vi "play-AFM-CS-imaging_v4.vi"() -> ()   [LabVIEW 2017]
uses:
  controls/boolean_info.ctl
  controls/TF-params.ctl
  controls/z-axis-params_v4_prescan.ctl
  <userlib>/_matio/level5/Public/MAT-File Data Types.ctl
  <vilib>/userdefined/High Color/nirio_resource_hc.ctl
  controls/expMetaData_prescan.ctl
  <vilib>/Utility/file.llb/Read Delimited Spreadsheet (DBL).vi
  <vilib>/FPGAPlugInAG/cRIO-9082/niLvFpga_Open_cRIO-9082.vi
  <vilib>/rvi/interface/common/dynamic/niFpgaDynamicAddResources.vi
  <vilib>/FPGAPlugInAG/Dynamic/niLvFpga_Reset_Dynamic.vi
  <vilib>/rvi/interface/common/niFpgaWaitOnOcc.vi
  <vilib>/Utility/error.llb/Error Cluster From Error Code.vi
  <vilib>/rvi/errors/niLvFpgaAdjustHostInterfaceError.vi
  <vilib>/FPGAPlugInAG/Dynamic/niLvFpga_Run_Dynamic.vi
  <vilib>/Utility/file.llb/Write Delimited Spreadsheet (DBL).vi
  <vilib>/FPGAPlugInAG/Dynamic/niLvFpga_Close_Dynamic.vi
  <userlib>/_matio/level5/Public/Write/Append Data Element.llb/Append Data Element (Anything).vi
  <vilib>/rvi/interface/nirviOpenFPGA/nirviOpenFPGA.xnode
  FPGA Bitfiles/afmimagingcontro_FPGATargetSPARTA_cs-scanningv4_7fR1l8pRFB8.lvbitx
  <vilib>/rvi/interface/nirviMethod/nirviMethod.xnode
  <vilib>/rvi/interface/nirviReadWriteControl/nirviReadWriteControl.xnode
  <vilib>/rvi/interface/nirviCloseFPGA/nirviCloseFPGA.xnode
  <vilib>/FPGAPlugInAG/Dynamic/niLvFpga_ConfigureFifo_Dynamic.vi
  <vilib>/rvi/errors/niLvFpgaMergeErrorWithErrorCode.vi
  <vilib>/rvi/interface/Simulation/niFpgaSimulationCallBeginRW.vi
  <vilib>/FPGAPlugInAG/Dynamic/niLvFpga_ReadFifo_Dynamic.vi
  NiFpgaLv.dll
  <userlib>/_matio/level5.lvlib
  fpga_interface_lib/fpga_interface.lvlib
panel:
  out "z-u(k)":sgl
  in  "do-Dz":bool
  in  "TF-params":T1={"TF-order"=2, "Num"=[1.0237086, -2.0434425, 1.0225973, 0.0, 0.0, 0.0, 0.0, 0.0, 0.0], "Den"=[1.0, -1.9961116, 0.998975, 0.0, 0.0, 0.0, 0.0, 0.0, 0.0]}
  in  "input-data-path":path
  out "boolean \nindicators":T2
  out "CS Time":dbl
  out "Current Case":i16
  out "state times":dbl[](array[numeric])
  out "entity-index":i16
  in  "Tab Control":T3(tab)
  in  "z_axis_params":T4={"TOL"=0.010000002, "z_u_max"=5.0, "setpoint-scan"=0.0, "Ki-scan"=0.02, "uz_safe"=0.0, "Kiz_down"=0.02, "prescan-samples"=500, "setpoint-up"=-0.3000030517578125} {"uz_safe" format="%#_13g"; "TOL" format="%#_13g"}
  in  "trigger-0":bool
  in  "numEntities":i16
  out "output-data-path":path
  out "output-meta-data-path":path
  in  "note-blob":string
  in  "overwrite":bool
  in  "TsTicks":u32=1600
  in  "Ki-xy":sgl=0.005
  in  "collect all":bool=TRUE
  in  "zup-err-threshold":fxp<+,24,5>=0.10000228881835938
  in  "xy settled-samples\n threshold":i16=200
  in  "xy error-threshold":sgl=0.01
  out "number-settled-samples-x":i16
  out "number-settled-samples-y":i16
  out "case-selected":i16
  out "number-settled-samples-Z":i16
  out "size(s)":i32
  out "nsamps":i32
  out "y iter":i32
  out "size(s) 2":i32[](array[numeric])
  out "Array":i32[][](array[numeric])
  out "error out 2":errorcluster
  out "z-control":dbl[](graph)
  out "x-axis":dbl[](graph)
  out "z-error":dbl[](graph)
  out "y-axis":dbl[](graph)
  in  "STOP":bool
  # "- If collect all = fasle and collect move = false,\nwe only collect measurement data.\n- If collect all = false, and collect move = true,\nwe collect measurement and move data.\n- If collect all = true, we collect everything."
  # "move"
  # "lower"
  # "z-settle"
  # "scan"
  # "tip-up"
  # "make this come from input csv!"
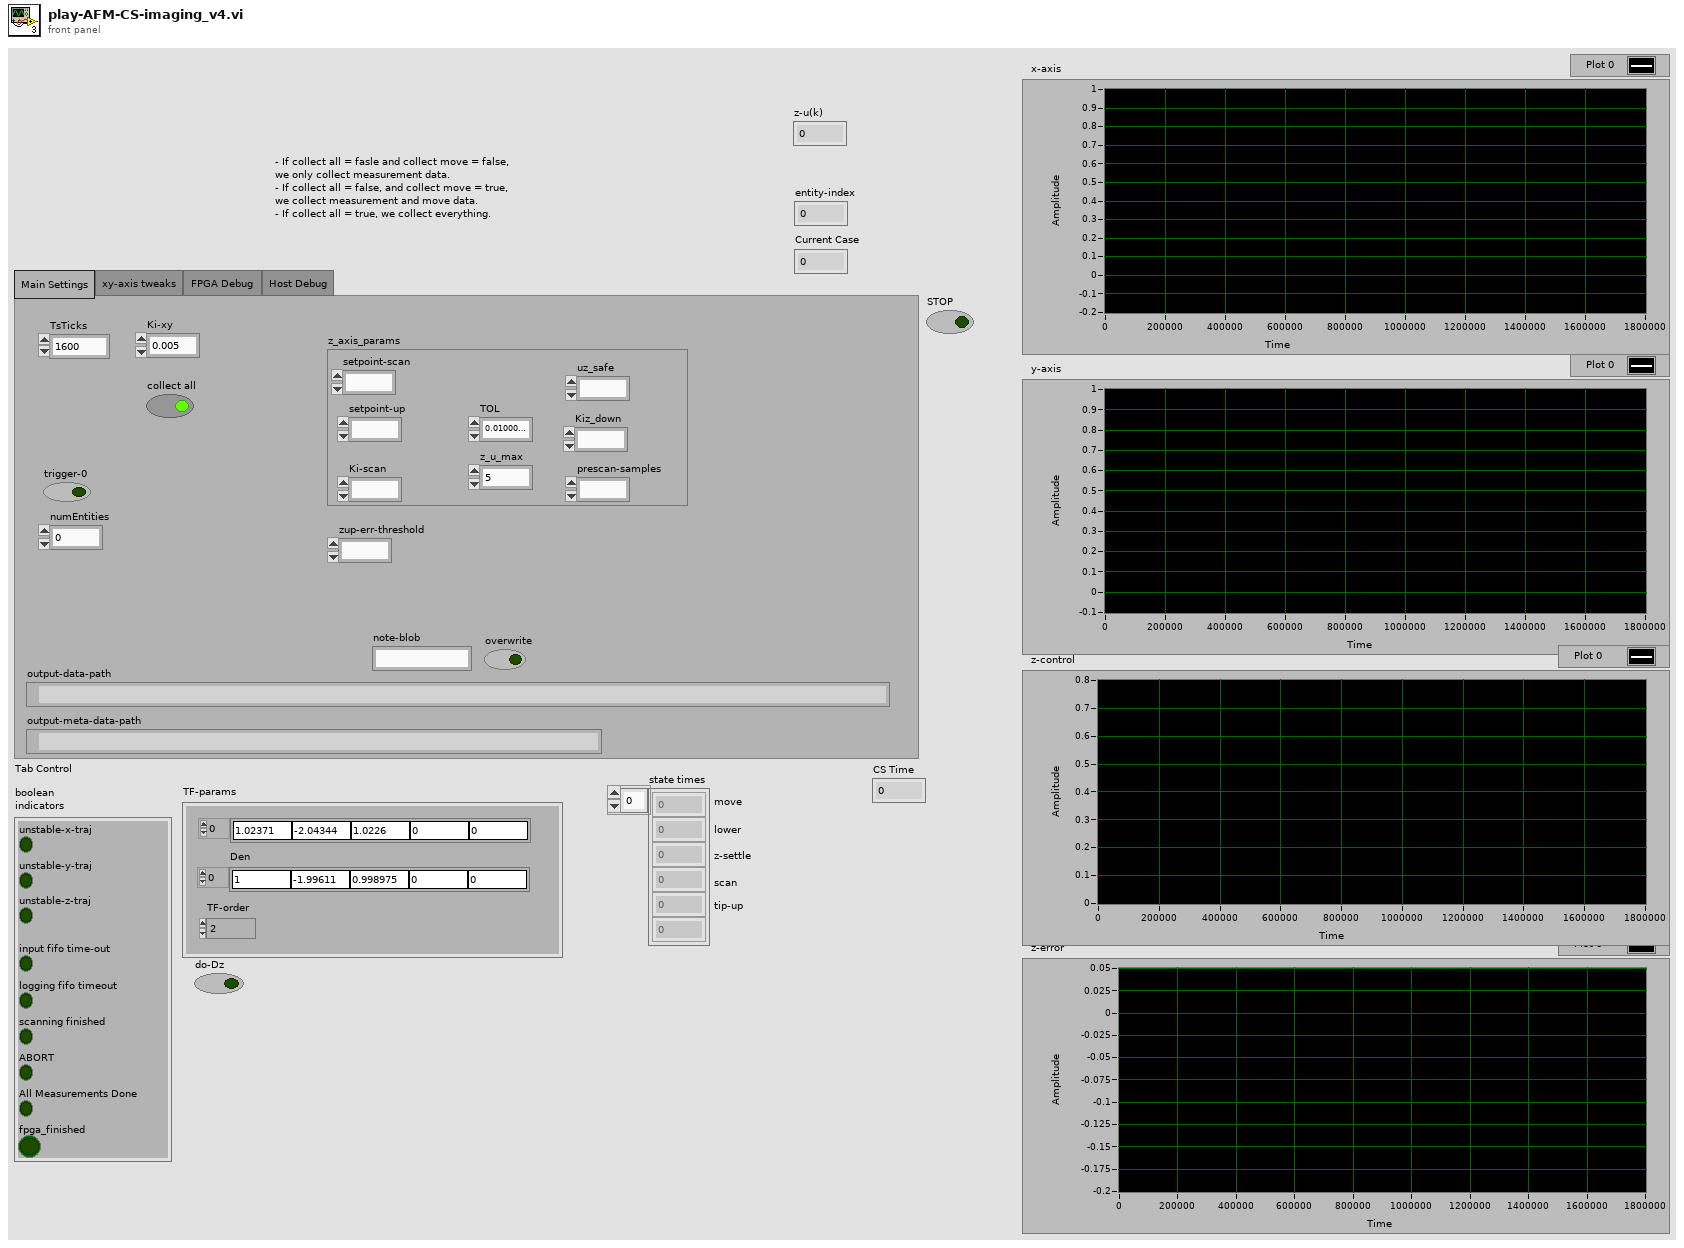
[diagram p1: front panel]
types:
  T1 = typedef "TF-params.ctl" = cluster{"TF-order":i16, "Num":sgl[], "Den":sgl[]}
  T2 = typedef "boolean_info.ctl" = cluster{"unstable-z-traj":bool, "input fifo time-out":bool, "logging fifo timeout":bool, "scanning finished":bool, "unstable-x-traj":bool, "unstable-y-traj":bool, "ABORT":bool, "All Measurements Done":bool, "fpga_finished":bool}
  T3 = enum32{"Main Settings", "xy-axis tweaks", "FPGA Debug ", "Host Debug"}
  T4 = typedef "z-axis-params_v4_prescan.ctl" = cluster{"TOL":sgl, "z_u_max":sgl, "setpoint-scan":fxp<+/-,32,16>, "Ki-scan":sgl, "uz_safe":fxp<+/-,16,5>, "Kiz_down":sgl, "prescan-samples":i16, "setpoint-up":fxp<+/-,32,16>}
  T5 = typedef "level5.lvlib/MAT-File Data Types.ctl" = enum32{"_invalid", "miINT8", "miUINT8", "miINT16", "miUINT16", "miINT32", "miUINT32", "miSINGLE", "_reserved_1", "miDOUBLE", "_reserved_2", "_reserved_3", "miINT64", "miUINT64", "miMATRIX", "miCOMPRESSED", "miUTF8", "miUTF16", "miUTF32"}
  T6 = typedef "nirio_resource_hc.ctl" = tag
  T7 = cluster{"unstable-z-traj":bool, "input fifo time-out":bool, "logging fifo timeout":bool, "scanning finished":bool, "unstable-x-traj":bool, "unstable-y-traj":bool, "ABORT":bool, "All Measurements Done":bool, "fpga_finished":bool}
  T8 = typedef "expMetaData_prescan.ctl" = cluster{"xy_error_threshold":sgl, "xy_settled_samples_threshold":i16, "Ki_xy":sgl, "state_counts":dbl[], "TOL":sgl, "z_u_max":sgl, "setpoint-up":sgl, "Ki-scan":sgl, "Z_error_threshold":sgl, "zup_N":i16, "Num":sgl[], "Den":sgl[], "prescan-samples":i16, "Kiz_down":sgl, "do_xy_CL":bool, "do_Alt_Ztrigger":bool, "output-data-path":path, "input-data-path":path, "zup-error-threshold":sgl, "setpoint-scan":sgl, "do_Dz":bool}
  T9 = enum16{"open", "replace", "create", "open or create", "replace or create", "replace or create with confirmation"}
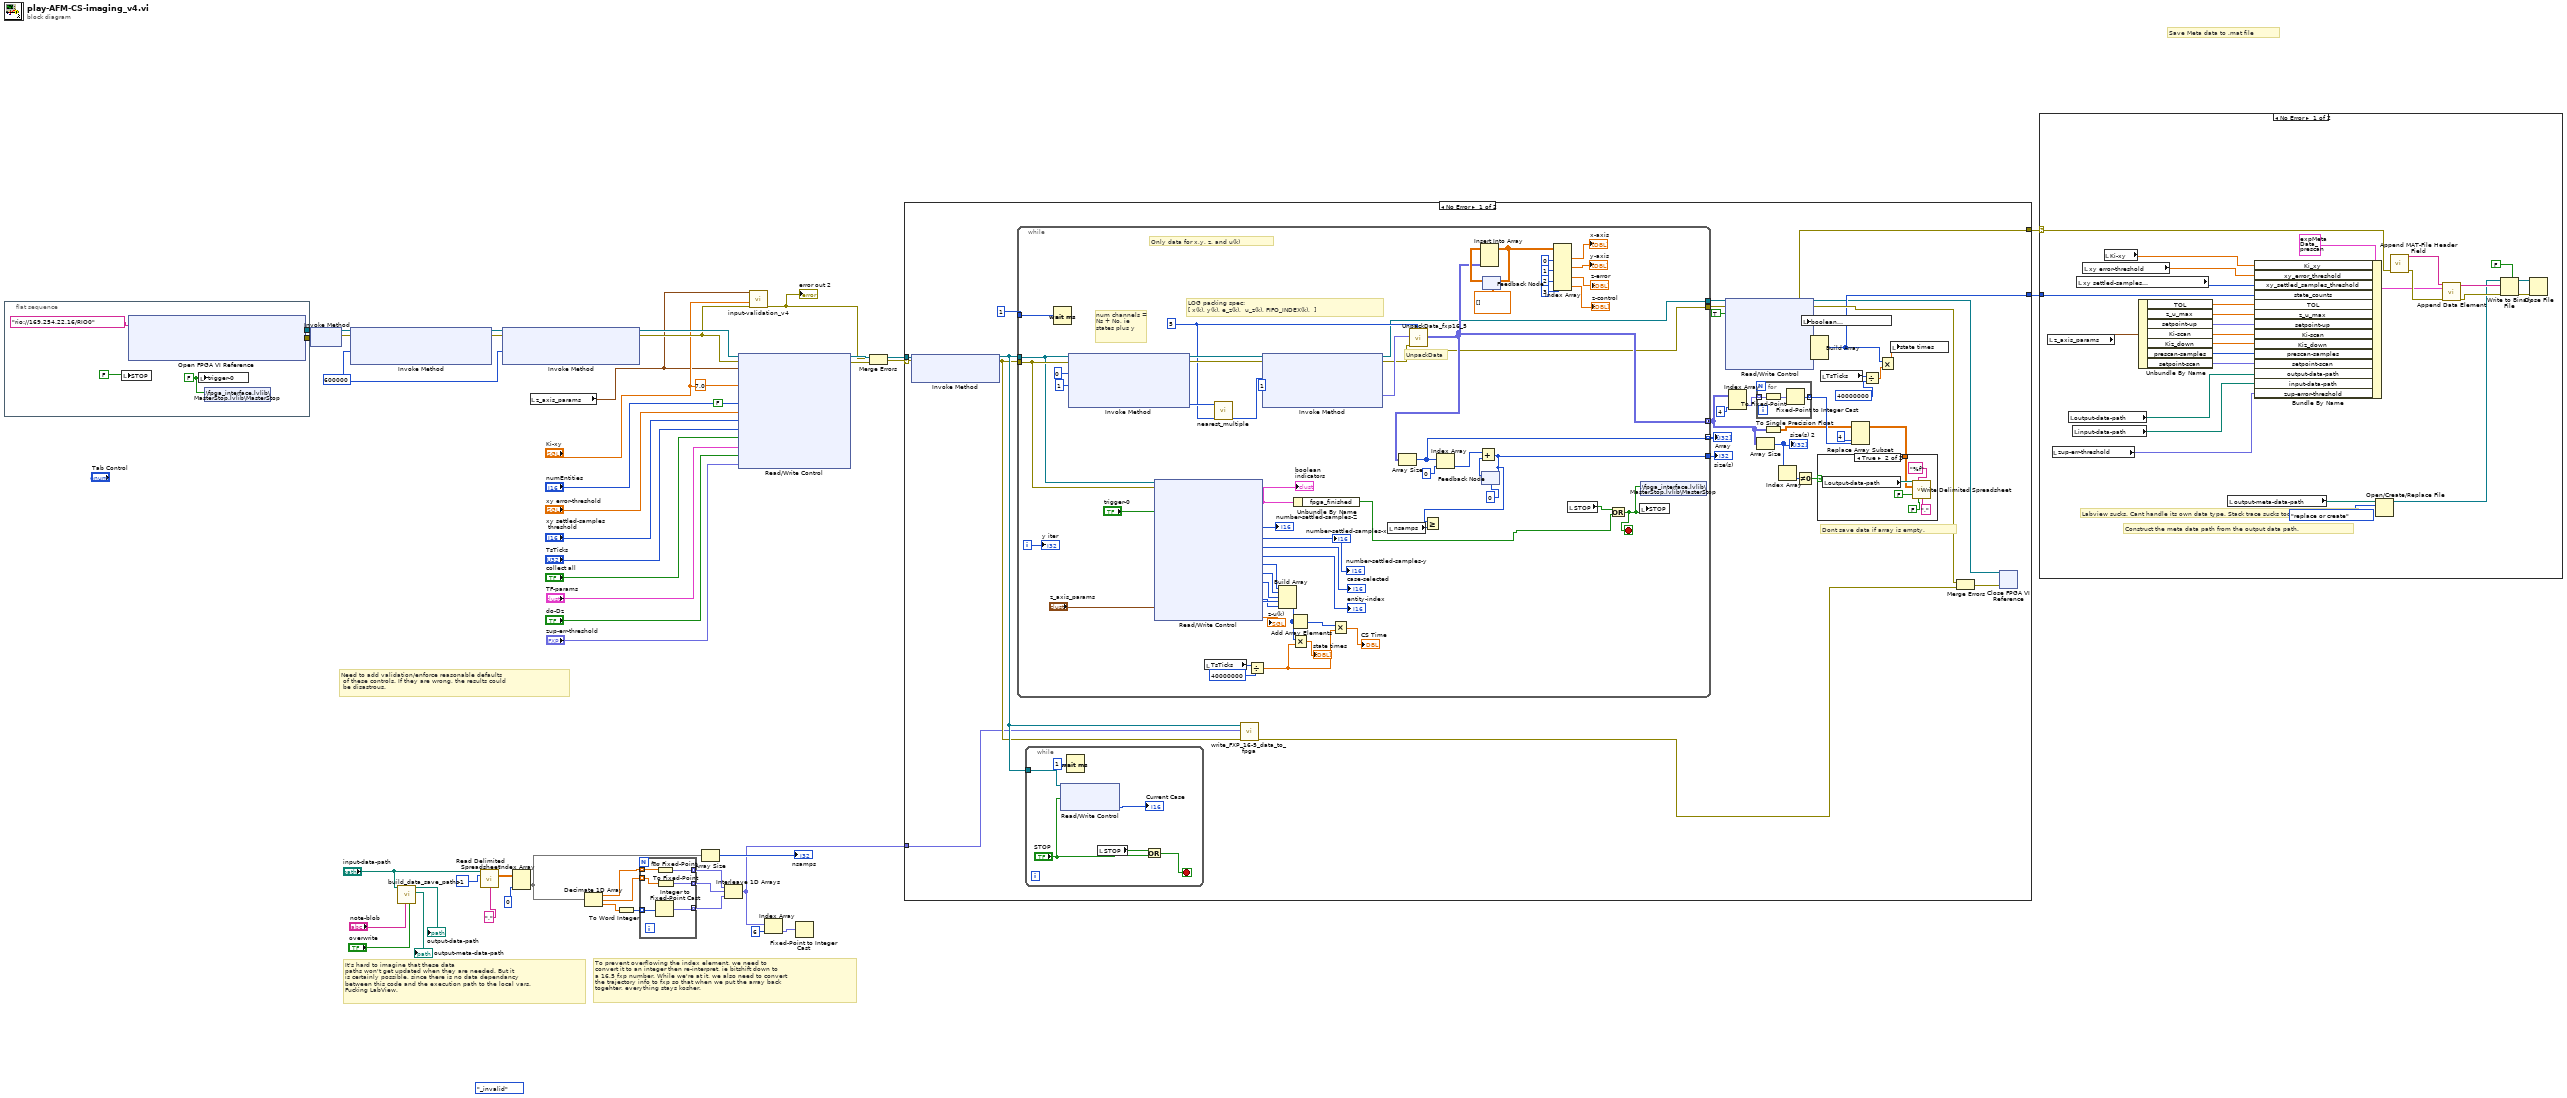
[diagram p0: block diagram]
diagram:
  (unwired) MAT-File_Data_Types."_invalid" ("MAT-File Data Types")
  w47 = 600000
  # "It's hard to imagine that these data\npaths won't get updated when they are needed. But it \nis certainly possible, since there is no data dependancy \nbetween this code and the execution path to the local vars.\nFucking LabView."
  # "Save Meta data to .mat file"
  # "To prevent overflowing the index element, we need to \nconvert it to an integer then re-interpret, ie bitshift down to \na 16,5 fxp number. While we're at it, we also need to convert\nthe trajectory info to fxp so that when we put the array back\ntogehter, everything stays kosher."
  # "Need to add validation/enforce reasonable defaults\n of these controls. If they are wrong, the results could\n be disastrous."
  n1 = flat-sequence {
    tunnel: [w53] -> w46
    tunnel: [w52] -> w45
    frame #0 {
      w49 = FALSE ("trigger-0")
      n2 = local write "STOP"(FALSE) -> ()
      n3 = xnode "Open FPGA VI Reference"("resource name"=T6 "rio://169.254.22.16/RIO0") -> ("FPGA VI Reference Out"=w53:refnum<k20>, "error out"=w52:errorcluster)  [unwired: 1 in]
      n4 = local write "trigger-0"(w49) -> ()
      n5 = shared-variable ".\\fpga_interface.lvlib\\MasterStop.lvlib\\MasterStop"(w49) -> ()  [unwired: 1 in, 1 out]
    }
  }
  n6 = xnode "Invoke Method"("FPGA VI Reference In"=w46, "error in"=w45) -> ("FPGA VI Reference Out"=w40:refnum<k20>, "error out"=w39:errorcluster)
  n7 = xnode "Invoke Method"("FPGA VI Reference In"=w40, "error in"=w39, "Requested Depth"=w47) -> ("FPGA VI Reference Out"=w42:refnum<k20>, "error out"=w43:errorcluster)  [unwired: 1 out]
  n8 = call "build_data_save_paths.vi"("overwrite"="overwrite", "note-blob"="note-blob", "input-file"="input-data-path") -> ("output-meta-data-path"=→"output-meta-data-path":path, "output-data-path"=→"output-data-path":path)  [unwired: 5 in, 2 out]
  n9 = call-poly <vilib>:"Read Delimited Spreadsheet.vi"("file path (dialog if empty)"="input-data-path", "number of rows (all:-1)"=-1, "delimiter (\\t)"=",") -> ("all rows"=w35:dbl[][])  [unwired: 7 in, 5 out]
  n10 = xnode "Invoke Method"("FPGA VI Reference In"=w42, "error in"=w43, "Requested Depth"=w47) -> ("FPGA VI Reference Out"=w48:refnum<k20>, "error out"=w5:errorcluster)  [unwired: 1 out]
  n11 = Index Array(array=w35, index (col)=0 ("dimension size")) -> (element=w18:dbl[])  [unwired: 1 in]
  n12 = local read "z_axis_params"() -> (w3:T4)
  n13 = Decimate 1D Array(w18) -> (w26:dbl[], w25:dbl[], w27:dbl[])
  n14 = To Word Integer(number=w27) -> (16bit integer=w24:i16[])
  n15 = for {
    tunnel: w26 -> [w59] mode=indexing
    tunnel: w25 -> [w58] mode=indexing
    tunnel: [w57] -> w22 mode=indexing
    tunnel: [w56] -> w23 mode=indexing
    tunnel: w24 -> [w55] mode=indexing
    tunnel: [w54] -> w21 mode=indexing
    n16 = Integer to Fixed-Point Cast(integer=w55) -> (fixed-point=w54:fxp<+/-,16,5>)  [unwired: 1 in]
    n17 = To Fixed-Point(number=w59) -> (fixed-point=w56:fxp<+/-,16,5>)  [unwired: 1 in]
    n18 = To Fixed-Point(number=w58) -> (fixed-point=w57:fxp<+/-,16,5>)  [unwired: 1 in]
  }
  n19 = Array Size(array=w18) -> (size(s)=→"nsamps":i32)
  n20 = Interleave 1D Arrays(w23, w22, w21) -> (w17:fxp<+/-,16,5>[])
  n21 = xnode "Read/Write Control"("FPGA VI Reference In"=w48, "error in"=w5, "z_axis_params"=w3, "xy-bound"=sgl 7.0, "Ki-xy"="Ki-xy", "trigger-0"=FALSE, "numEntities"="numEntities", "xy-error-threshold"="xy error-threshold", "settled-samples threshold"="xy settled-samples\n threshold", "TsTicks"="TsTicks", "collect all"="collect all", "TF-params"="TF-params", "do-Dz"="do-Dz", "zup-err-threshold"="zup-err-threshold") -> ("FPGA VI Reference Out"=w41:refnum<k20>, "error out"=w28:errorcluster)
  n22 = call "input-validation_v4.vi"("error constant"=w5, "Ki-xy"="Ki-xy", "z_axis_params"=w3) -> ("error out"=w6:errorcluster)  [unwired: 8 in]
  "error out 2" <- w6
  n23 = Index Array(array=w17, index=6) -> (element=w20:fxp<+/-,16,5>)
  n24 = Fixed-Point to Integer Cast(1:w20) -> ()  [unwired: 1 out]
  n25 = Merge Errors(w6, w28) -> (w9:errorcluster)
  n26 = case shown="No Error" w9 {
    selector: w9 -> [w64 w169]
    tunnel: w41 -> [w95 _]
    tunnel: w17 -> [w61 _]
    tunnel: [w94 w169] -> w15
    tunnel: [w93 _] -> w14
    frame No Error {
      # "Dont save data if array is empty."
      n27 = xnode "Invoke Method"("FPGA VI Reference In"=w95, "error in"=w64) -> ("FPGA VI Reference Out"=w63:refnum<k20>, "error out"=w62:errorcluster)  [unwired: 1 in]
      n28 = while {
        tunnel: 1 -> [w168]
        tunnel: w63 -> [w156]
        tunnel: w62 -> [w157]
        tunnel: [w127] -> w89
        tunnel: [w134] -> w80 mode=concatenating
        tunnel: [w154] -> w91
        tunnel: [w132] -> w88
        tunnel: [w149] -> w85 mode=indexing
        i -> [w155]
        stop <- w111 stop-if-true
        w135 = u32 5 ("y")
        # "LOG packing spec:\n[ x(k), y(k), e_z(k),  u_z(k), FIFO_INDEX(k),  ]"
        # "num channels = Ns + No, ie states plus y"
        # "Only data for x,y, z, and u(k)"
        # "UnpackData"
        n29 = Wait (ms)(milliseconds to wait=w168) -> ()  [unwired: 1 out]
        n30 = xnode "Invoke Method"("FPGA VI Reference In"=w156, "error in"=w157, "Number of Elements"=0 ("Timeout (ms)"), "Timeout (ms)"=1) -> ("FPGA VI Reference Out"=w164:refnum<k20>, "error out"=w165:errorcluster, "Elements Remaining"=w152:u32)  [unwired: 1 out]
        n31 = xnode "Read/Write Control"("FPGA VI Reference In"=w156, "error in"=w157, "trigger-0"="trigger-0", "z_axis_params"="z_axis_params") -> ("boolean  indicators"=w120:T7, "number-settled-samples-Z"=→"number-settled-samples-Z":i16, "number-settled-samples-x"=→"number-settled-samples-x":i16, "number-settled-samples-y"=→"number-settled-samples-y":i16, "Current Case"=→"case-selected":u8, "entity-index"=→"entity-index":i16, "state1-count"=w116:u64, "state2-count"=w115:u64, "state3-count"=w114:u64, "state4-count"=w129:u64, "state5-count"=w128:u64, "z-u(k)"=→"z-u(k)":sgl)  [unwired: 1 in, 2 out]
        "boolean \nindicators" <- w120
        n32 = local read "TsTicks"() -> (w123:u32)
        n33 = call "nearest_multiple.vi"("numChan"=w135, "N"=w152) -> ("(int) y*floor(x/y)"=w151:u64)  [unwired: 9 in]
        n34 = Divide(x=w123, y=u32 40000000) -> (x/y=w118:dbl)
        n35 = xnode "Invoke Method"("FPGA VI Reference In"=w164, "error in"=w165, "Number of Elements"=w151, "Timeout (ms)"=1) -> ("FPGA VI Reference Out"=w127:refnum<k20>, "error out"=w132:errorcluster, "Data"=w133:fxp<+/-,16,5>[])  [unwired: 1 out]
        n36 = Build Array(w116, w115, w114, w129, w128) -> (w119:u64[])
        n37 = Add Array Elements(numeric array=w119) -> (sum=w124:u64)
        n38 = Multiply(x=w119, y=w118) -> (x*y=→"state times":dbl[])
        n39 = Unbundle By Name(w120) -> ("fpga_finished"=w131:bool)
        n40 = Multiply(x=w124, y=w118) -> (x*y=→"CS Time":dbl)
        n41 = local read "nsamps"() -> (w161:i32)
        n42 = call "UnpackData_fxp16_5.vi"("NumChannels"=w135, "error In"=w132, "1D Data In"=w133) -> ("2D Data Out"=w134:fxp<+/-,16,5>[][])  [unwired: 7 in, 1 out]
        n43 = Array Size(array=w134) -> (size(s)=w149:i32[])
        n44 = Index Array(array=w149, index=0) -> (element=w159:i32)
        n45 = feedback #1(0) -> (w160:i32)
        n46 = Add(x=w159, y=w160) -> (x+y=w154:i32)
        n47 = Greater Or Equal?(x=w154, y=w161) -> ()  [unwired: 1 out]
        n48 = feedback-in #1(w154) -> ()
        n49 = feedback #2(dbl[][] []) -> (w145:dbl[][])
        n50 = Insert Into Array(array=w145, new element=w134) -> (w136:dbl[][])  [unwired: 2 in]
        n51 = feedback-in #2(w136) -> ()
        n52 = Index Array(array=w136, index (col) #1=0 ("disabled index (col)"), index (col) #2=1 ("index (col)"), index (col) #3=2 ("index (col)"), index (col) #4=3 ("index (col)")) -> (element #1=→"x-axis":dbl[], element #2=→"y-axis":dbl[], element #3=→"z-error":dbl[], element #4=→"z-control":dbl[])  [unwired: 4 in]
        n53 = local read "STOP"() -> (w150:bool)
        n54 = Or(x=w150, y=w131) -> (x .or. y?=w111:bool)
        n55 = local write "STOP"(w111) -> ()
        n56 = shared-variable ".\\fpga_interface.lvlib\\MasterStop.lvlib\\MasterStop"(w111) -> ()  [unwired: 1 in, 1 out]
        "y iter" <- w155
      }
      "size(s)" <- w91
      "Array" <- w85
      n57 = while {
        tunnel: w63 -> [w110]
        stop <- w106 stop-if-true
        n58 = xnode "Read/Write Control"("FPGA VI Reference In"=w110, "ABORT"="STOP") -> ("Current Case"=→"Current Case":u8)  [unwired: 1 in, 2 out]
        n59 = Wait (ms)(milliseconds to wait=u32 1) -> ()  [unwired: 1 out]
        n60 = local read "STOP"() -> (w107:bool)
        n61 = Or(x=w107, y="STOP") -> (x .or. y?=w106:bool)
      }
      n62 = call "write_FXP_16-5_data_to_fpga.vi"("error in"=w62, "all rows"=w61, "FPGA Interface"=w63) -> ("error out"=w60:errorcluster)  [unwired: 7 in, 1 out]
      n63 = xnode "Read/Write Control"("FPGA VI Reference In"=w89, "error in"=w88, "ABORT"=TRUE) -> ("FPGA VI Reference Out"=w86:refnum<k20>, "error out"=w94:errorcluster, "boolean  indicators"=w69:T7, "state1-count"=w78:u64, "state2-count"=w77:u64, "state3-count"=w76:u64, "state4-count"=w75:u64, "state5-count"=w74:u64)
      n64 = Index Array(array=w80, index (col)=4) -> (element=w83:fxp<+/-,16,5>[])  [unwired: 1 in]
      n65 = for {
        tunnel: w83 -> [w103] mode=indexing
        tunnel: [w104] -> w81 mode=indexing
        n66 = To Fixed-Point(number=w103) -> (fixed-point=w102:fxp<+/-,16,5>)  [unwired: 1 in]
        n67 = Fixed-Point to Integer Cast(1:w102) -> (0:w104:i16)
      }
      n68 = Array Size(array=w80) -> (size(s)=w70:i32[])
      "size(s) 2" <- w70
      n69 = To Single Precision Float(number=w80) -> (single precision float=w79:sgl[][])
      n70 = Index Array(array=w70) -> (element=w71:i32)  [unwired: 1 in]
      n71 = Not Equal To 0?(x=w71) -> (x != 0?=w72:bool)
      n72 = local write "boolean \nindicators"(w69) -> ()
      n73 = Build Array(w78, w77, w76, w75, w74) -> (w93:u64[])
      n74 = local read "TsTicks"() -> (w68:u32)
      n75 = Replace Array Subset(array=w79, new element=w81, index (col)=4) -> (w73:sgl[][])  [unwired: 1 in]
      n76 = case shown="True" w72 {
        tunnel: w73 -> [_ w96]
        frame False {
        }
        frame True {
          n77 = local read "output-data-path"() -> (w101:path)
          n78 = call-poly <vilib>:"Write Delimited Spreadsheet.vi"("file path (dialog if empty)"=w101, "format (%.3f)"="%f", "2D data"=w96, "append to file? (new file:F)"=FALSE, "transpose? (no:F)"=FALSE, "delimiter (\\t)"=",") -> ()  [unwired: 8 in, 2 out]
        }
      }
      n79 = Divide(x=w68, y=u32 40000000) -> (x/y=w66:dbl)
      n80 = Multiply(x=w93, y=w66) -> (x*y=w65:dbl[])
      n81 = local write "state times"(w65) -> ()
      n82 = Merge Errors(w94, w60) -> (w90:errorcluster)
      n83 = xnode "Close FPGA VI Reference"("FPGA VI Reference In"=w86, "error in"=w90) -> ()  [unwired: 1 out]
    }
    frame Error {
    }
  }
  n84 = case shown="No Error" w15 {
    selector: w15 -> [w190 _]
    tunnel: w14 -> [w184 _]
    frame No Error {
      # "Construct the meta data path from the output data path."
      # "Labview sucks. Cant handle its own data type. Stack trace sucks too."
      n85 = local read "z_axis_params"() -> (w183:T4)
      n86 = local read "zup-err-threshold"() -> (w170:fxp<+,24,5>)
      n87 = local read "output-data-path"() -> (w176:path)
      n88 = local read "input-data-path"() -> (w177:path)
      n89 = local read "xy settled-samples\n threshold"() -> (w180:i16)
      n90 = local read "xy error-threshold"() -> (w181:sgl)
      n91 = local read "Ki-xy"() -> (w182:sgl)
      n92 = Unbundle By Name(w183) -> ("TOL"=w187:sgl, "z_u_max"=w186:sgl, "setpoint-up"=w174:fxp<+/-,32,16>, "Ki-scan"=w185:sgl, "Kiz_down"=w173:sgl, "prescan-samples"=w171:i16, "setpoint-scan"=w172:fxp<+/-,32,16>)
      n93 = local read "output-meta-data-path"() -> (w178:path)
      n94 = Bundle By Name(cluster=T8 {"xy_error_threshold"=0.1, "xy_settled_samples_threshold"=200, "Ki_xy"=0.005, "state_counts"=[], "TOL"=0.3, "z_u_max"=5.0, "setpoint-up"=-5e-06, "Ki-scan"=0.001, "Z_error_threshold"=0.0, "zup_N"=5000, "Num"=[-0.00254, 0.000408, 0.00295, 0.0, 0.0, 0.0, 0.0, 0.0, 0.0], "Den"=[0.982758, -1.98194, 1.0, 0.0, 0.0, 0.0, 0.0, 0.0, 0.0], "prescan-samples"=0, "Kiz_down"=0.001, "do_xy_CL"=FALSE, "do_Alt_Ztrigger"=FALSE, "output-data-path"=path "", "input-data-path"=path "", "zup-error-threshold"=0.0, "setpoint-scan"=0.0, "do_Dz"=FALSE} ("ExpMetaData"), "Ki_xy"=w182, "xy_error_threshold"=w181, "xy_settled_samples_threshold"=w180, "state_counts"=w184, "TOL"=w187, "z_u_max"=w186, "setpoint-up"=w174, "Ki-scan"=w185, "Kiz_down"=w173, "prescan-samples"=w171, "setpoint-scan"=w172, "output-data-path"=w176, "input-data-path"=w177, "zup-error-threshold"=w170) -> (w188:T8)
      n95 = Open/Create/Replace File(file path (use dialog)=w178, operation (0:open)=T9."replace or create") -> (refnum out=w189:refnum<file>)  [unwired: 4 in, 2 out]
      n96 = call <userlib>:"Append MAT-File Header Field.vi"("error"=w190) -> ("result string"=w197:string, "error out"=w191:errorcluster)  [unwired: 13 in]
      n97 = call-poly <userlib>:"Append Data Element.vi"("initial string"=w197, "data"=w188, "error in (no error)"=w191) -> ("result string"=w195:string, "error out"=w196:errorcluster)  [unwired: 11 in]
      n98 = Write to Binary File(file (use dialog)=w189, data=w195, error in=w196, 5:FALSE ("prepend array or string size? (T)")) -> (refnum out=w192:refnum<file>, error out=w193:errorcluster)  [unwired: 2 in, 1 out]
      n99 = Close File(refnum=w192, error in=w193) -> ()  [unwired: 2 out]
    }
    frame Error {
    }
  }
